vi "Generic command handler.vi"(8 "error in (no error)":errorcluster, 10 "Message in":refnum<class "GenericMessage.lvclass">, 11 "Template in":refnum<class "Template.lvclass">) -> (0 "error out":errorcluster, 2 "value":string, 3 "Template out":refnum<class "Template.lvclass">)   [LabVIEW 2012, in "Template.lvclass"]
doc: "The generic_command_handler processes the command 'generic'. Commands which are not part of the predefined list of commands fall under the 'generic' command for special activity."
uses:
  Template.lvclass
  <vilib>/Distrio/Murmex/GenericMessage/GenericMessage.lvclass
  <vilib>/Distrio/Murmex/Murmex/Murmex.lvclass
  <vilib>/measure/NI_MABase.lvlib
panel:
  out "Waveform Graph":waveform(dbl)(graph)
  # "This method is called when the GENERIC\ntrigger is sent. \n\nOverride this method when your component needs to\nrespond to this trigger. \n\nCall parent for proper implementation"
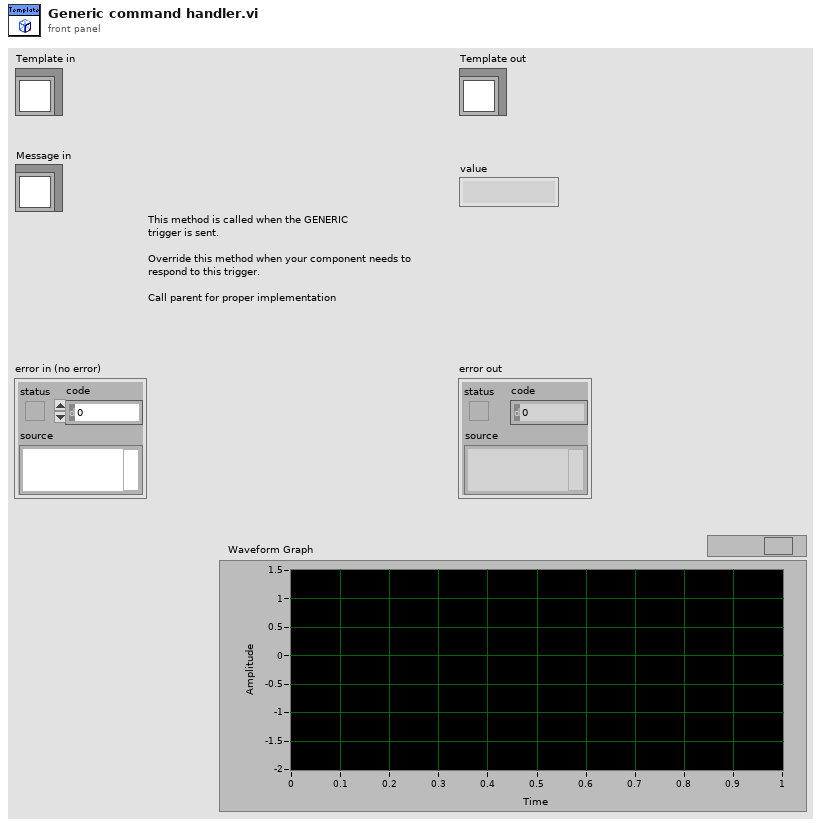
[diagram p1: front panel]
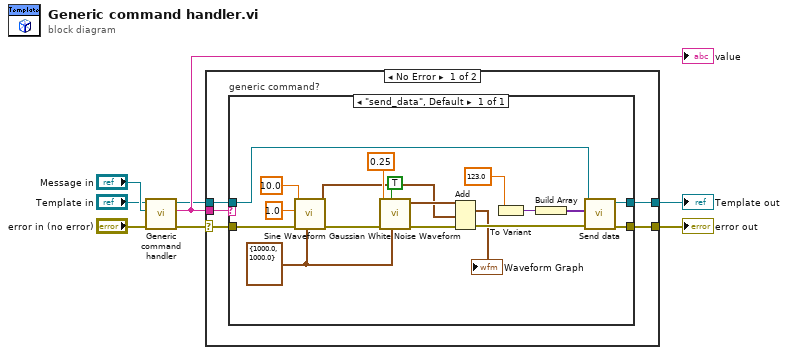
[diagram p0: block diagram]
diagram:
  n1 = call-parent "Generic command handler.vi"("error in (no error)"="error in (no error)", "Message in"="Message in", "Murmex in"="Template in") -> ("error out"=w5:errorcluster, "value"=w3:string, "Murmex out"=w2:refnum<class "Template.lvclass">)  [unwired: 6 in]
  "value" <- w3
  n2 = case shown="No Error" w5 {
    selector: w5 -> [w10 w33]
    tunnel: [w11 w33] -> w4
    tunnel: w3 -> [w13 _]
    tunnel: w2 -> [w12 w32]
    tunnel: [w9 w32] -> w1
    frame No Error {
      n3 = case "generic command?" shown="\"send_data\", Default" w13 {
        tunnel: w12 -> [w19]
        tunnel: [w20] -> w11
        tunnel: w10 -> [w31]
        tunnel: [w18] -> w9
        frame "send_data", Default {
          w22 = cluster{"Fs":dbl, "#s":dbl} {"Fs"=1000.0, "#s"=1000.0} ("sampling info")
          n4 = call <vilib>:"Sine Waveform.vi"("sampling info"=w22, "error in (no error)"=w31, "amplitude"=1.0, "frequency"=10.0) -> ("error out"=w28:errorcluster, "signal out"=w25:waveform(dbl))  [unwired: 6 in]
          n5 = call <vilib>:"Gaussian White Noise Waveform.vi"("sampling info"=w22, "reset signal"=TRUE, "error in (no error)"=w28, "standard deviation"=0.25) -> ("error out"=w24:errorcluster, "signal out"=w26:waveform(dbl))  [unwired: 6 in]
          n6 = Add(1:w25, 2:w26, 4:w24) -> (0:→"Waveform Graph":waveform(dbl), 3:w23:errorcluster)
          n7 = To Variant(anything=123.0) -> (Variant=w16:variant)
          n8 = Build Array(w16) -> (w15:variant[])
          n9 = call <vilib>:"Send data.vi"("error in (no error)"=w23, "data (channels array)"=w15, "Murmex in"=w19) -> ("error out"=w20:errorcluster, "Murmex out"=w18:refnum<class "Template.lvclass">)  [unwired: 7 in]
        }
      }
    }
    frame Error {
    }
  }
  "error out" <- w4
  "Template out" <- w1
